vi "Shooter Controller.vi"(8 "error in":errorcluster) -> ()   [LabVIEW 2025]
doc: "This VI executes continuously carrying out the current operation and responding to updates or new operations. It will often contain the timing or control code that is difficult to place directly in TeleOp. This VI generally opens all sensors and motors and isolates the rest of the robot code from knowing how the operations are carried out."
uses:
  <vilib>/Rock Robotics/WPI/Framework/Completion Status.ctl
  Shooter Setpoints.ctl
  Shooter Operations.ctl
  <vilib>/Rock Robotics/WPI/ThirdParty/REV Robotics/REVLib/Typedef/SPARK Feed Forward Gains.ctl
  <vilib>/Rock Robotics/WPI/ThirdParty/REV Robotics/REVLib/Typedef/Spark MAX Idle Mode.ctl
  <vilib>/Rock Robotics/WPI/ThirdParty/REV Robotics/REVLib/Typedef/Spark MAX Control Type.ctl
  a9f37026-b6b8-4123-ad44-c3b165350157.vi
  c75955a9-db3f-439f-a07d-65bfe6422968.vi
  3a433730-1b2e-4c17-a59a-3af33b5bd4e0.vi
  <vilib>/Rock Robotics/WPI/ThirdParty/REV Robotics/REVLib/SubVI/Public/SPARK Open Brushless.vi
  <vilib>/Rock Robotics/WPI/ThirdParty/REV Robotics/REVLib/SubVI/Public/SPARK Configure Basic Idle Mode.vi
  Framework/Robot Global Data.vi
  <vilib>/Rock Robotics/WPI/ThirdParty/REV Robotics/REVLib/SubVI/Public/SPARK Get Encoder Status Velocity.vi
  <vilib>/Rock Robotics/Network Tables/NT Write Boolean.vi
panel:
  in  "Kicker Gains":T2={{"P Gain"=0.0002, "I Gain"=0.0, "D Gain"=0.005}, "Feed Forward Gains"={"kV"=0.00181, "kS"=0.0, "kA"=0.0, "kG"=0.0, "kCos"=0.0, "kCosRatio"=0.0}, "I Zone"=0.0, "Min Output"=-0.95, "Max Output"=0.95}
  out "Kicker PID graph":T3(graph)={"Kicker Setpoint"=0.0, "Sensor Velocity"=-0.005231584422290325}
  in  "Flywheel PID":T2={{"P Gain"=0.00045, "I Gain"=0.0, "D Gain"=0.04}, "Feed Forward Gains"={"kV"=0.0018, "kS"=0.0, "kA"=0.0, "kG"=0.0, "kCos"=0.0, "kCosRatio"=0.0}, "I Zone"=0.0, "Min Output"=-0.95, "Max Output"=0.95}
  in  "Hood Gains":T2={{"P Gain"=0.00019999999999999998, "I Gain"=0.0, "D Gain"=0.005}, "Feed Forward Gains"={"kV"=0.00196, "kS"=0.0, "kA"=0.0, "kG"=0.0, "kCos"=0.0, "kCosRatio"=0.0}, "I Zone"=0.0, "Min Output"=-0.95, "Max Output"=0.95}
  out "Hood PID graph":T4(graph)={"Hood Setpoint"=5000.0, "Sensor Velocity"=5015.6142578125}
  out "Flywheel PID graph":T5(graph)={"Flywheel Setpoint"=1000.0, "Sensor Velocity"=980.640869140625}
  in  "Interactive Values":T6
  out "Current\nCmd":string="Started at  00:14:15.362\nDefault: Reserve,  S 0.0, D 0.000000"
  in  "Buttons":cluster{"Execute Cmd":bool, "Abort Cmd":bool}
  out "Command Timing":cluster{"Start Time (ms)":u32, "Iterations":i32}={"Start Time (ms)"=933391, "Iterations"=0}
  out "Status":T8
  # "Interactive Command: You may fill in the settings for a command\nand schedule it with the Execute button. You can observe and abort\nany command while fine tuning the code for the controller."
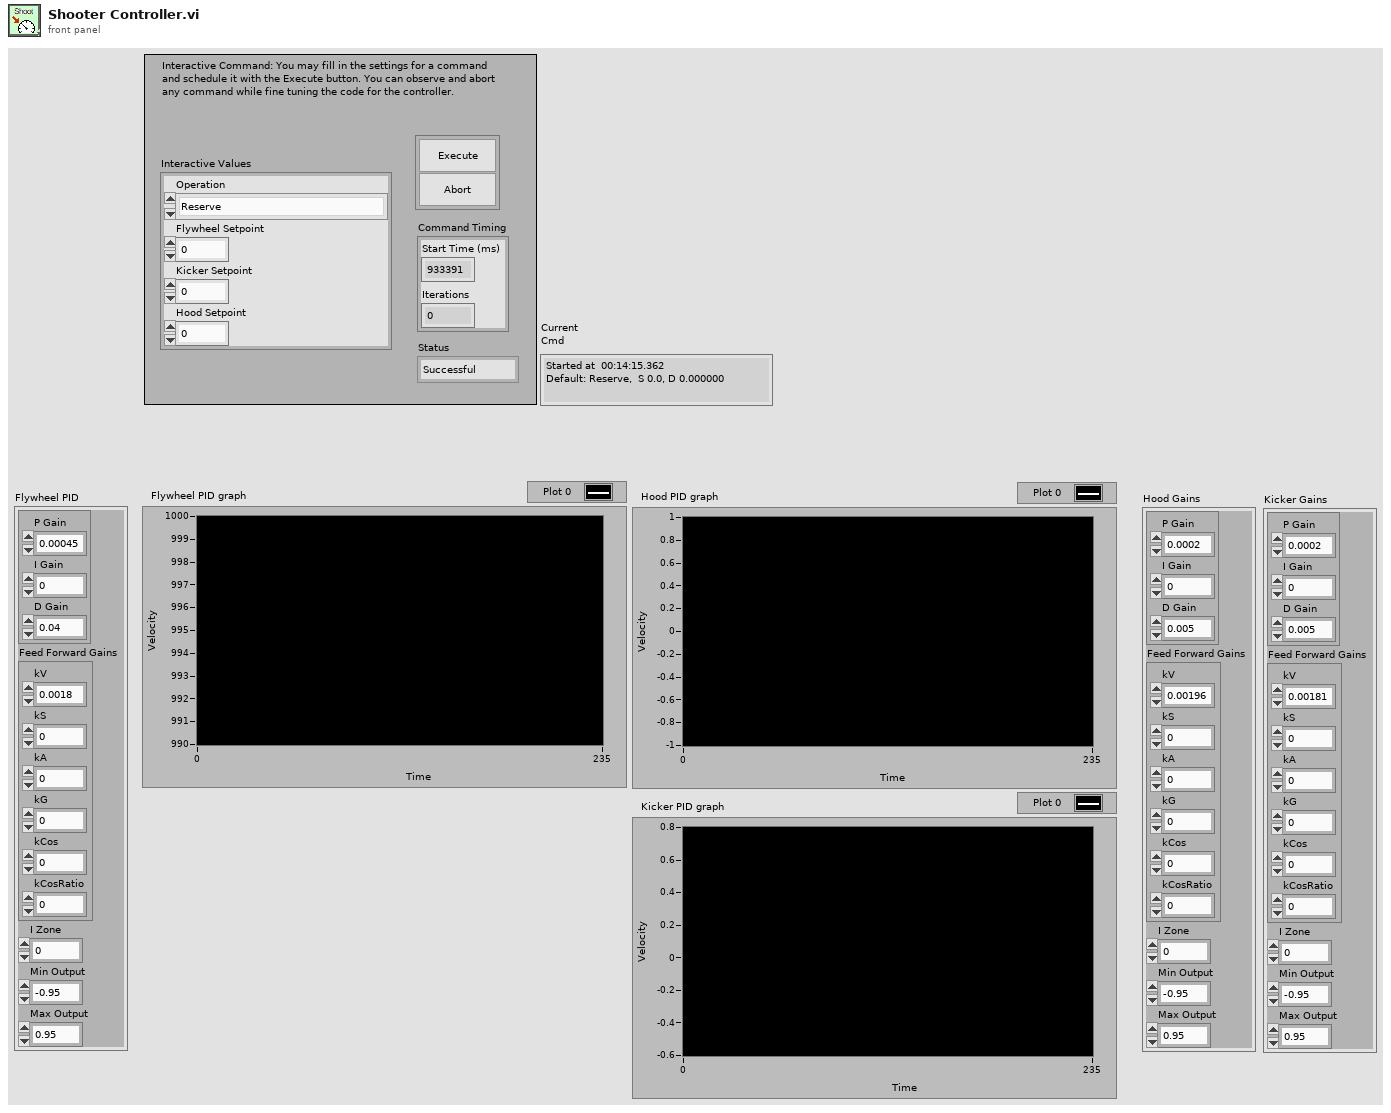
[diagram p1: front panel]
types:
  T1 = typedef "SPARK Feed Forward Gains.ctl" = cluster{"kV":dbl, "kS":dbl, "kA":dbl, "kG":dbl, "kCos":dbl, "kCosRatio":dbl}
  T2 = cluster{cluster{"P Gain":dbl, "I Gain":dbl, "D Gain":dbl}, "Feed Forward Gains":T1, "I Zone":dbl, "Min Output":dbl, "Max Output":dbl}
  T3 = cluster{"Kicker Setpoint":dbl, "Sensor Velocity":dbl}
  T4 = cluster{"Hood Setpoint":dbl, "Sensor Velocity":dbl}
  T5 = cluster{"Flywheel Setpoint":dbl, "Sensor Velocity":dbl}
  T6 = typedef "Shooter Setpoints.ctl" = cluster{"Operation":T7, "Flywheel Setpoint":dbl, "Kicker Setpoint":dbl, "Hood Setpoint":dbl}
  T7 = typedef "Shooter Operations.ctl" = enum16{"Reserve", "Read Current", "Immediate", "Interpolated Shot"}
  T8 = typedef "Completion Status.ctl" = enum16{"Successful", "Aborted", "Incomplete"}
  T9 = typedef "Spark MAX Idle Mode.ctl" = enum16{"Coast", "Brake"}
  T10 = typedef "WPI_MotorControlDeviceRef.ctl" = cluster{"DeviceStatus":errorcluster, "Type":T11, "PWM":cluster{"PWM Channel":T12, "DeadBand":T13}, "CAN":cluster{"Device Number":u8, "SetOutput VI Ref":variant, "GetOutput VI Ref":variant, "Enable VI Ref":variant, "Disable VI Ref":variant, "Data":variant}, "Invert":bool, "DIO PWM":cluster{"PWM \"Enable\" Channel":T12, "DIOChannel":T14, "PWM Rate":dbl}}
  T11 = typedef "WPI_MotorControlType.ctl" = enum16{"PWM", "CAN", "DIO PWM"}
  T12 = typedef "FPGA_DIOPWMChannel.ctl" = enum8{"PWM 0", "PWM 1", "PWM 2", "PWM 3", "PWM 4", "PWM 5", "PWM 6", "PWM 7", "PWM 8", "PWM 9", "PWM MXP 0", "PWM MXP 1", "PWM MXP 2", "PWM MXP 3", "PWM MXP 4", "PWM MXP 5", "PWM MXP 6", "PWM MXP 7", "PWM MXP 8", "PWM MXP 9", "Invalid"}
  T13 = typedef "WPI_PWMDeadband.ctl" = cluster{"Name":string, "maxPositivePwm":i32, "minPositivePwm":i32, "centerPwm":i32, "maxNegativePwm":i32, "minNegativePwm":i32, "angularRange":u16}
  T14 = typedef "FPGA_DIOChannel.ctl" = enum8{"DIO 0", "DIO 1", "DIO 2", "DIO 3", "DIO 4", "DIO 5", "DIO 6", "DIO 7", "DIO 8", "DIO 9", "DIO MXP 0", "DIO MXP 1", "DIO MXP 2", "DIO MXP 3", "DIO MXP 4", "DIO MXP 5", "DIO MXP 6", "DIO MXP 7", "DIO MXP 8", "DIO MXP 9", "DIO MXP 10", "DIO MXP 11", "DIO MXP 12", "DIO MXP 13", "DIO MXP 14", "DIO MXP 15", "SPI Port CS1", "SPI Port CS2", "SPI Port CS3", "SPI Port MISO", "SPI Port MOSI", "Invalid"}
  T15 = typedef "Command Status Info.ctl" = cluster{"Name":string, "Status":T8, "notifier out":T16}
  T16 = typedef "Completion Notifier.ctl" = refnum<notifier>
  T17 = cluster{"Current Command":T6, "Command Timing":cluster{"Start Time (ms)":u32, "Iterations":i32}, "Command Arguments":cluster{"Command Info":T15, "Description":string, "Default Command":T6, "queue out":refnum<queue>, "Subsystem Name":string}}
  T18 = typedef "Spark MAX Control Type.ctl" = enum16{"Percent VBus", "Voltage", "Velocity", "Position", "Smart Motion", "Current", "Smart Velocity", "MAXMotion Position", "MAXMotion Velocity"}
  T19 = cluster{"Follower Ref":T10, "Shooter Ref":T10, "MotorControlDeviceRef out":T10, "MotorControlDeviceRef out":T10}
  T20 = typedef "WPI_DriverStationRobotMode2.ctl" = enum16{"Autonomous Disabled", "Autonomous Enabled", "Teleop Disabled", "Teleop Enabled", "Disconnected", "Finish", "Test Disabled", "Test Enabled", "Emergency Stopped"}
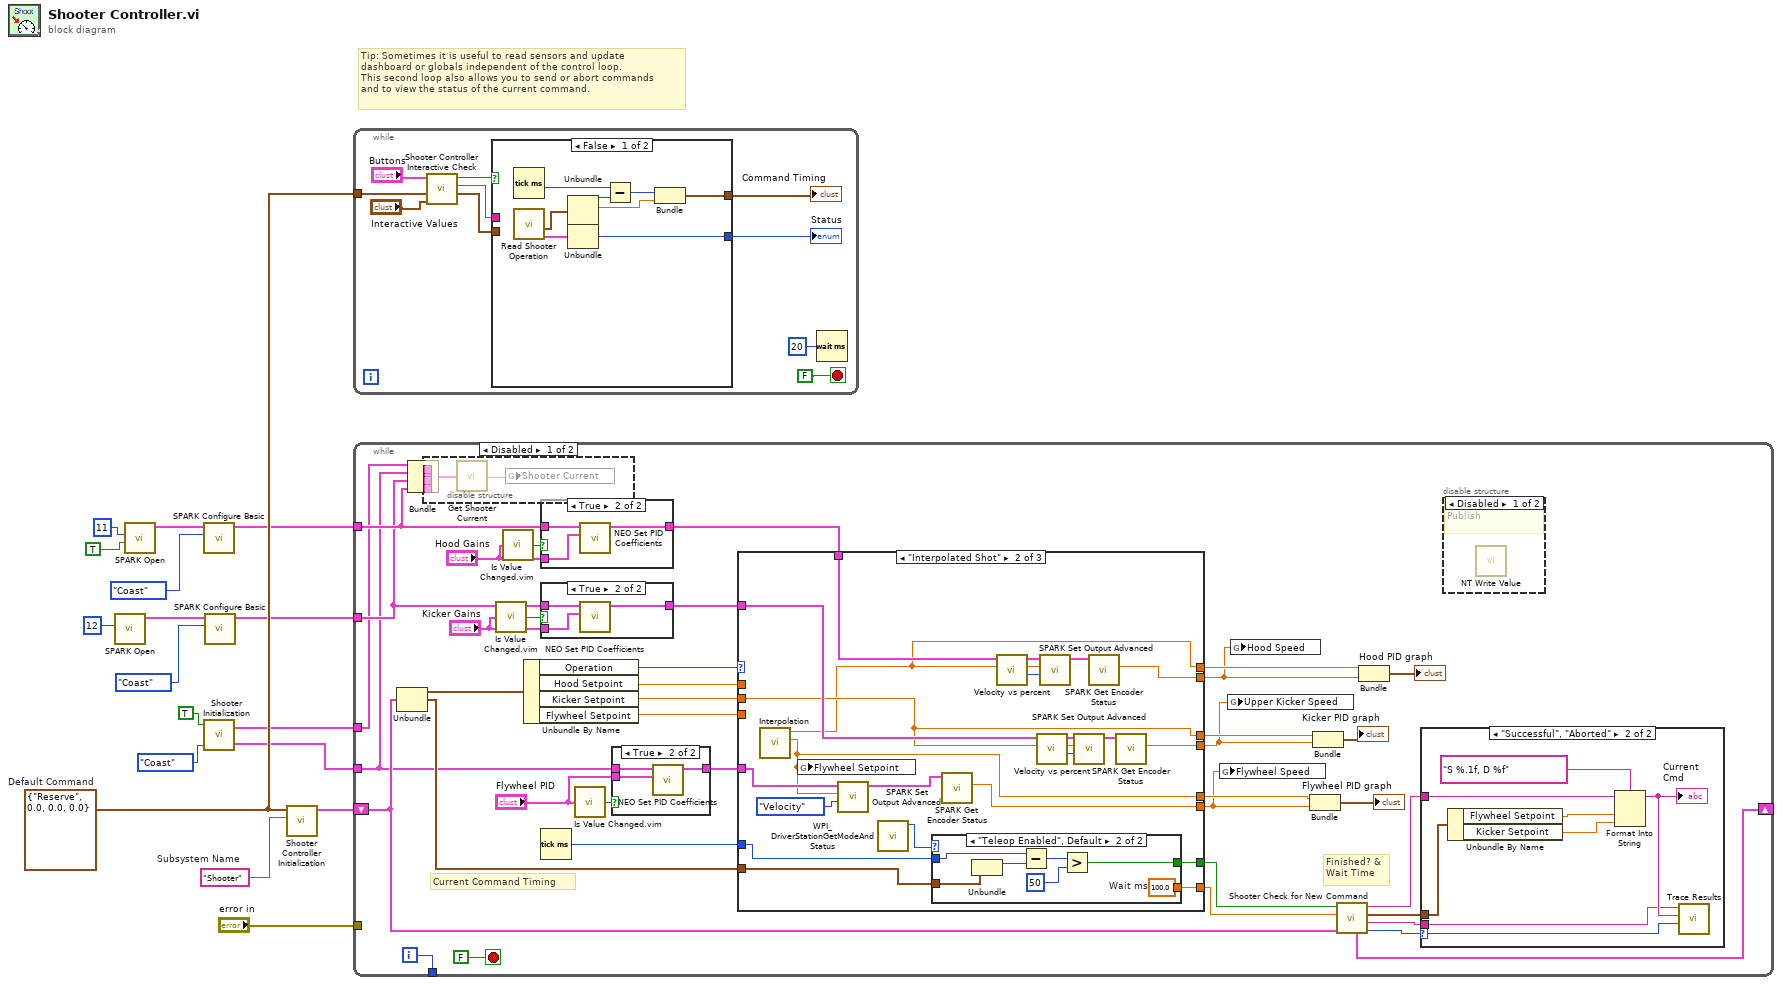
[diagram p0: block diagram]
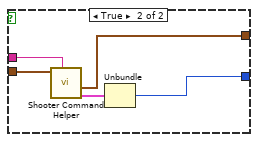
[diagram p2: hidden frame]
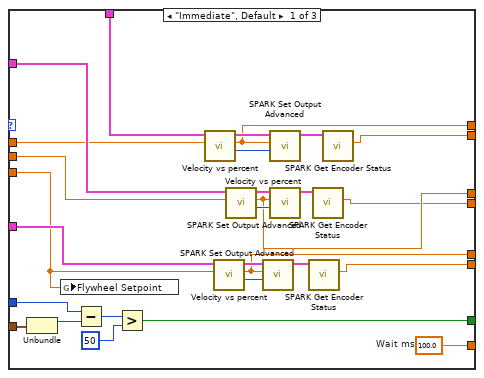
[diagram p9: hidden frame]
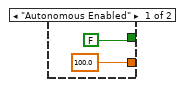
[diagram p10: hidden frame]
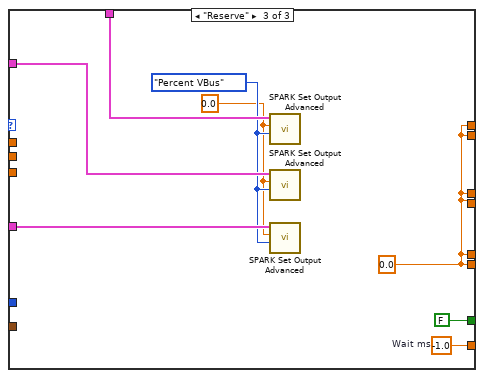
[diagram p11: hidden frame]
diagram:
  w14 = T6 {"Operation"=enum."Reserve", "Flywheel Setpoint"=0.0, "Kicker Setpoint"=0.0, "Hood Setpoint"=0.0}  # Default Command
  w15 = "Shooter"  # Subsystem Name
  # "Tip: Sometimes it is useful to read sensors and update\ndashboard or globals independent of the control loop.\nThis second loop also allows you to send or abort commands\nand to view the status of the current command."
  n1 = call-poly <vilib>:"SPARK Open.vi"("Device Number"=u8 12) -> ("MotorControlDeviceRef"=w5:T10)  [unwired: 9 in, 1 out]
  n2 = call-poly <vilib>:"SPARK Open.vi"("Invert"=TRUE, "Device Number"=u8 11) -> ("MotorControlDeviceRef"=w12:T10)  [unwired: 8 in, 1 out]
  n3 = call-poly <vilib>:"SPARK Configure Basic.vi"("Idle Mode"=Spark_MAX_Idle_Mode."Coast", "MotorControlDeviceRef in"=w12) -> ("MotorControlDeviceRef out"=w11:T10)  [unwired: 8 in, 1 out]
  n4 = call "Shooter Initialization.vi"("Idle Mode"=Spark_MAX_Idle_Mode."Coast", "Invert Follower"=TRUE) -> ("Shooter Ref"=w2:T10, "Follower Ref"=w1:T10)  [unwired: 1 in]
  n5 = call-poly <vilib>:"SPARK Configure Basic.vi"("Idle Mode"=Spark_MAX_Idle_Mode."Coast", "MotorControlDeviceRef in"=w5) -> ("MotorControlDeviceRef out"=w3:T10)  [unwired: 8 in, 1 out]
  n6 = call "Shooter Controller Initialization.vi"("Subsystem Name"=w15, "Default Command"=w14) -> ("Current Command"=w16:T17)  [unwired: 9 in]
  n7 = while {
    tunnel: w14 -> [w24]
    stop <- FALSE stop-if-true
    n8 = call "Shooter Controller Interactive Check.vi"("Interactive Command in"="Interactive Values", "Default Command"=w24, "Buttons"="Buttons") -> ("Interactive Command out"=w21:T6, "Trace String"=w22:string, "Schedule"=w23:bool)  [unwired: 6 in]
    n9 = case shown="False" w23 {
      tunnel: [w35 w40] -> w20
      tunnel: w21 -> [_ w38]
      tunnel: [w31 w36] -> w19
      tunnel: w22 -> [_ w39]
      frame False {
        n10 = Tick Count (ms)() -> (millisecond timer value=w30:u32)
        n11 = call "Read Shooter Operation.vi"() -> ("Command Info"=w28:T15, "SubSystem Data"=w29:T6)  [unwired: 9 in, 1 out]
        n12 = Unbundle(w29) -> ("Operation"=w34:T7, "Flywheel Setpoint"=w32:dbl)  [unwired: 2 out]
        n13 = Unbundle(w28) -> ("Status"=w35:T8)  [unwired: 2 out]
        n14 = Subtract(x=w30, y=w34) -> (x-y=w33:u32)
        n15 = Bundle(w33, "Flywheel Setpoint"=w32) -> (w31:cluster{u32, "Flywheel Setpoint":dbl})  [unwired: 1 in]
      }
      frame True {
        n16 = call "Shooter Command Helper.vi"("Description"=w39, "SubSystem Data"=w38) -> ("Command Info Out"=w37:T15, "Command Timing"=w36:cluster{"Start Time (ms)":u32, "Iterations":i32})  [unwired: 7 in, 1 out]
        n17 = Unbundle(w37) -> ("Status"=w40:T8)  [unwired: 2 out]
      }
    }
    "Status" <- w20
    "Command Timing" <- w19
    n18 = Wait (ms)(milliseconds to wait=u32 20) -> ()  [unwired: 1 out]
  }
  n19 = while {
    shift-right: [w73] -> _
    shift-left: w16 -> [w66]
    tunnel: [w78] -> _
    tunnel: "error in" -> [_]
    tunnel: w11 -> [w47]
    tunnel: w2 -> [w45]
    tunnel: w3 -> [w46]
    tunnel: w1 -> [w44]
    i -> [w78]
    stop <- FALSE stop-if-true
    # "Current Command Timing"
    # "Finished? &\nWait Time"
    n20 = Unbundle(w66) -> ("Current Command"=w77:T6, "Command Timing"=w75:cluster{"Start Time (ms)":u32, "Iterations":i32})  [unwired: 1 out]
    n21 = disable-structure shown="Disabled" {
      disable-tunnel: w47 -> [w85 _]
      disable-tunnel: w46 -> [w84 _]
      disable-tunnel: w45 -> [w83 _]
      disable-tunnel: w44 -> [w82 _]
      frame Disabled {
        n22 = Bundle("Follower Ref"=w82, "Shooter Ref"=w83, "MotorControlDeviceRef out"=w84, "MotorControlDeviceRef out"=w85) -> (w81:T19)  [unwired: 1 in]
        n23 = call "Get Shooter Current.vi"("Motors in"=w81) -> ("Total Current"=w80:dbl)
        n24 = global write "Robot Global Data.vi" "Shooter Current"(w80) -> ()
      }
      frame Enabled {
      }
    }
    n25 = call "Is Value Changed.vim"("value"="Kicker Gains") -> ("changed or first call?"=w55:bool)
    n26 = call "Is Value Changed.vim"("value"="Hood Gains") -> ("changed or first call?"=w60:bool)
    n27 = Unbundle By Name(w77) -> ("Operation"=w54:T7, "Hood Setpoint"=w74:dbl, "Kicker Setpoint"=w63:dbl, "Flywheel Setpoint"=w62:dbl)
    n28 = case shown="True" w60 {
      tunnel: w47 -> [w94 w97]
      tunnel: [w94 w96] -> w65
      tunnel: "Hood Gains" -> [_ w95]
      frame False {
      }
      frame True {
        n29 = call "NEO Set PID Coefficients.vi"("Drive PID Gains"=w95, "MotorControlDeviceRef in"=w97) -> ("MotorControlDeviceRef out"=w96:T10)  [unwired: 6 in, 1 out]
      }
    }
    n30 = case shown="True" w55 {
      tunnel: w46 -> [w86 w89]
      tunnel: [w86 w88] -> w57
      tunnel: "Kicker Gains" -> [_ w87]
      frame False {
      }
      frame True {
        n31 = call "NEO Set PID Coefficients.vi"("Drive PID Gains"=w87, "MotorControlDeviceRef in"=w89) -> ("MotorControlDeviceRef out"=w88:T10)  [unwired: 6 in, 1 out]
      }
    }
    n32 = Tick Count (ms)() -> (millisecond timer value=w76:u32)
    n33 = call "Is Value Changed.vim"("value"="Flywheel PID") -> ("changed or first call?"=w58:bool)
    n34 = case shown="True" w58 {
      tunnel: w45 -> [w90 w93]
      tunnel: [w90 w92] -> w64
      tunnel: "Flywheel PID" -> [_ w91]
      frame False {
      }
      frame True {
        n35 = call "NEO Set PID Coefficients.vi"("Drive PID Gains"=w91, "MotorControlDeviceRef in"=w93) -> ("MotorControlDeviceRef out"=w92:T10)  [unwired: 6 in, 1 out]
      }
    }
    n36 = case shown="\"Interpolated Shot\"" w54 {
      tunnel: [w133 w151 w174] -> w71
      tunnel: [w127 w152 FALSE] -> w72
      tunnel: w75 -> [w129 w153 _]
      tunnel: w76 -> [w128 w154 _]
      tunnel: w74 -> [w112 _ _]
      tunnel: w65 -> [w113 w147 w173]
      tunnel: w57 -> [w117 w143 w172]
      tunnel: w64 -> [w121 w156 w171]
      tunnel: w63 -> [w116 w137 _]
      tunnel: w62 -> [w120 _ _]
      tunnel: [w111 w137 w167] -> w50
      tunnel: [w110 w138 w167] -> w42
      tunnel: [w109 w140 w167] -> w49
      tunnel: [w108 w141 w167] -> w41
      tunnel: [w107 w134 w167] -> w48
      tunnel: [w106 w135 w167] -> w43
      frame "Immediate", Default {
        w133 = 100.0  # Wait ms
        n37 = Unbundle(w129) -> ("Start Time (ms)"=w132:u32)  [unwired: 1 out]
        n38 = global write "Robot Global Data.vi" "Flywheel Setpoint"(w120) -> ()
        n39 = Subtract(x=w128, y=w132) -> (x-y=w131:u32)
        n40 = Greater?(x=w131, y=u8 50 ("Left Motor")) -> (0:w127:bool)
        n41 = call "Velocity vs percent.vi"("Value in"=w112, "MotorControlDeviceRef in"=w113) -> ("Mode out"=w114:T18, "Value out"=w107:dbl, "MotorControlDeviceRef out"=w115:T10)  [unwired: 7 in]
        n42 = call "Velocity vs percent.vi"("Value in"=w120, "MotorControlDeviceRef in"=w121) -> ("Mode out"=w122:T18, "Value out"=w109:dbl, "MotorControlDeviceRef out"=w123:T10)  [unwired: 7 in]
        n43 = call "Velocity vs percent.vi"("Value in"=w116, "MotorControlDeviceRef in"=w117) -> ("Mode out"=w118:T18, "Value out"=w111:dbl, "MotorControlDeviceRef out"=w119:T10)  [unwired: 7 in]
        n44 = call <vilib>:"SPARK Set Output Advanced.vi"("Control Mode"=w122, "Setpoint"=w109, "MotorControlDevRef"=w123) -> ("MotorControlDevRef"=w125:T10)  [unwired: 7 in, 1 out]
        n45 = call <vilib>:"SPARK Set Output Advanced.vi"("Control Mode"=w114, "Setpoint"=w107, "MotorControlDevRef"=w115) -> ("MotorControlDevRef"=w126:T10)  [unwired: 7 in, 1 out]
        n46 = call <vilib>:"SPARK Set Output Advanced.vi"("Control Mode"=w118, "Setpoint"=w111, "MotorControlDevRef"=w119) -> ("MotorControlDevRef"=w124:T10)  [unwired: 7 in, 1 out]
        n47 = call-poly <vilib>:"SPARK Get Encoder Status.vi"("MotorControlDevRef in"=w125) -> ("Sensor Velocity"=w108:dbl)  [unwired: 7 in, 3 out]
        n48 = call-poly <vilib>:"SPARK Get Encoder Status.vi"("MotorControlDevRef in"=w124) -> ("Sensor Velocity"=w110:dbl)  [unwired: 7 in, 3 out]
        n49 = call-poly <vilib>:"SPARK Get Encoder Status.vi"("MotorControlDevRef in"=w126) -> ("Sensor Velocity"=w106:dbl)  [unwired: 7 in, 3 out]
      }
      frame "Interpolated Shot" {
        n50 = call "Interpolation.vi"() -> ("Flywheel Interp"=w140:dbl, "Hood Interp"=w134:dbl)  [unwired: 6 in]
        n51 = global write "Robot Global Data.vi" "Flywheel Setpoint"(w140) -> ()
        n52 = call <vilib>:"SPARK Set Output Advanced.vi"("Control Mode"=Spark_MAX_Control_Type."Velocity", "Setpoint"=w140, "MotorControlDevRef"=w156) -> ("MotorControlDevRef"=w142:T10)  [unwired: 7 in, 1 out]
        n53 = call <vilib>:"WPI_DriverStationGetModeAndStatus.vi"() -> ("Robot Mode"=w155:T20)  [unwired: 10 in, 1 out]
        n54 = case shown="\"Teleop Enabled\", Default" w155 {
          tunnel: [100.0 ("Wait ms") w166] -> w151
          tunnel: w153 -> [_ w162]
          tunnel: w154 -> [_ w160]
          tunnel: [FALSE w161] -> w152
          frame "Autonomous Enabled" {
          }
          frame "Teleop Enabled", Default {
            w166 = 100.0  # Wait ms
            n55 = Unbundle(w162) -> ("Start Time (ms)"=w165:u32)  [unwired: 1 out]
            n56 = Subtract(x=w160, y=w165) -> (x-y=w164:u32)
            n57 = Greater?(x=w164, y=u8 50 ("Left Motor")) -> (0:w161:bool)
          }
        }
        n58 = call-poly <vilib>:"SPARK Get Encoder Status.vi"("MotorControlDevRef in"=w142) -> ("Sensor Velocity"=w141:dbl)  [unwired: 7 in, 3 out]
        n59 = call "Velocity vs percent.vi"("Value in"=w134, "MotorControlDeviceRef in"=w147) -> ("Mode out"=w148:T18, "Value out"=w149:dbl, "MotorControlDeviceRef out"=w150:T10)  [unwired: 7 in]
        n60 = call "Velocity vs percent.vi"("Value in"=w137, "MotorControlDeviceRef in"=w143) -> ("Mode out"=w144:T18, "Value out"=w145:dbl, "MotorControlDeviceRef out"=w146:T10)  [unwired: 7 in]
        n61 = call <vilib>:"SPARK Set Output Advanced.vi"("Control Mode"=w148, "Setpoint"=w149, "MotorControlDevRef"=w150) -> ("MotorControlDevRef"=w136:T10)  [unwired: 7 in, 1 out]
        n62 = call <vilib>:"SPARK Set Output Advanced.vi"("Control Mode"=w144, "Setpoint"=w145, "MotorControlDevRef"=w146) -> ("MotorControlDevRef"=w139:T10)  [unwired: 7 in, 1 out]
        n63 = call-poly <vilib>:"SPARK Get Encoder Status.vi"("MotorControlDevRef in"=w136) -> ("Sensor Velocity"=w135:dbl)  [unwired: 7 in, 3 out]
        n64 = call-poly <vilib>:"SPARK Get Encoder Status.vi"("MotorControlDevRef in"=w139) -> ("Sensor Velocity"=w138:dbl)  [unwired: 7 in, 3 out]
      }
      frame "Reserve" {
        w167 = 0.0 ("Hood Interp")
        w168 = 0.0 ("Setpoint")
        w169 = Spark_MAX_Control_Type."Percent VBus" ("Control Mode")
        w174 = -1.0  # Wait ms
        n65 = call <vilib>:"SPARK Set Output Advanced.vi"("Control Mode"=w169, "Setpoint"=w168, "MotorControlDevRef"=w173) -> ()  [unwired: 7 in, 2 out]
        n66 = call <vilib>:"SPARK Set Output Advanced.vi"("Control Mode"=w169, "Setpoint"=w168, "MotorControlDevRef"=w172) -> ()  [unwired: 7 in, 2 out]
        n67 = call <vilib>:"SPARK Set Output Advanced.vi"("Control Mode"=w169, "Setpoint"=w168, "MotorControlDevRef"=w171) -> ()  [unwired: 7 in, 2 out]
      }
    }
    n68 = global write "Robot Global Data.vi" "Flywheel Speed"(w41) -> ()
    n69 = global write "Robot Global Data.vi" "Upper Kicker Speed"(w42) -> ()
    n70 = global write "Robot Global Data.vi" "Hood Speed"(w43) -> ()
    n71 = Bundle("Hood Interp"=w49, "Hood Interp"=w41) -> (→"Flywheel PID graph":cluster{"Hood Interp":dbl, "Hood Interp":dbl})  [unwired: 1 in]
    n72 = Bundle("Hood Interp"=w50, "Hood Interp"=w42) -> (→"Kicker PID graph":cluster{"Hood Interp":dbl, "Hood Interp":dbl})  [unwired: 1 in]
    n73 = call "Shooter Check for New Command.vi"("Current Command"=w66, "Wait time (ms)"=w71, "Finished?"=w72) -> ("Completion"=w67:T8, "Subsystem Name"=w68:string, "Current Command"=w69:T6, "Initial Trace String"=w70:string, "NextCommand"=w73:T17)  [unwired: 4 in]
    n74 = Bundle("Hood Interp"=w48, "Hood Interp"=w43) -> (→"Hood PID graph":cluster{"Hood Interp":dbl, "Hood Interp":dbl})  [unwired: 1 in]
    n75 = case shown="\"Successful\", \"Aborted\"" w67 {
      selector: w67 -> [_ w105]
      tunnel: w70 -> [_ w101]
      tunnel: w69 -> [_ w102]
      tunnel: w68 -> [_ w98]
      frame "Incomplete", Default {
        # "Continuing current command"
      }
      frame "Successful", "Aborted" {
        # "Report and setup for next command"
        n76 = Unbundle By Name(w102) -> ("Flywheel Setpoint"=w104:dbl, "Kicker Setpoint"=w99:dbl)
        n77 = Format Into String(format string="S %.1f, D %f", initial string=w101, w104, w99) -> (resulting string=w100:string)  [unwired: 1 in, 1 out]
        "Current\nCmd" <- w100
        n78 = call <vilib>:"Trace Results.vi"("Status of previous command"=w105, "Description"=w100, "Subsystem"=w98) -> ()  [unwired: 9 in]
      }
    }
    n79 = disable-structure shown="Disabled" {
      frame Disabled {
        # "Publish"
        n80 = call-poly <vilib>:"NT Write Value.vi"() -> ()  [unwired: 11 in, 1 out]
      }
      frame Enabled {
      }
    }
  }
